vi "divide.vi"(8 "error in (no error)":errorcluster, 9 "divisor":refnum<class "Image.lvclass">, 10 "divisor":dbl=1.0, 11 "Image in":refnum<class "Image.lvclass">) -> (0 "error out":errorcluster, 3 "Image out":refnum<class "Image.lvclass">)   [LabVIEW 2010, in "Image.lvclass"]
uses:
  Image.lvclass
  storage_mode.ctl
  ErrorController/ErrorController/class_data.vi
  <vilib>/vision/NI_Vision_Development_Module.lvlib
  ErrorController/ErrorController/ErrorController.lvclass
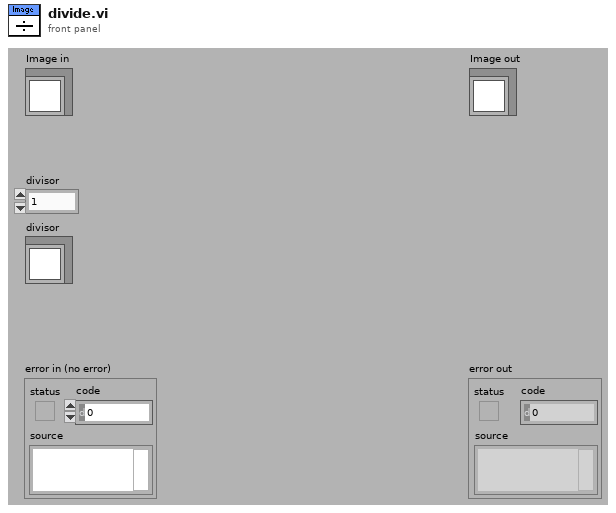
[diagram p1: front panel]
types:
  T1 = typedef "Image.lvclass/storage_mode.ctl" = enum16{"RAM", "disk"}
  T2 = typedef "IMAQ Image.ctl" = refnum<image>
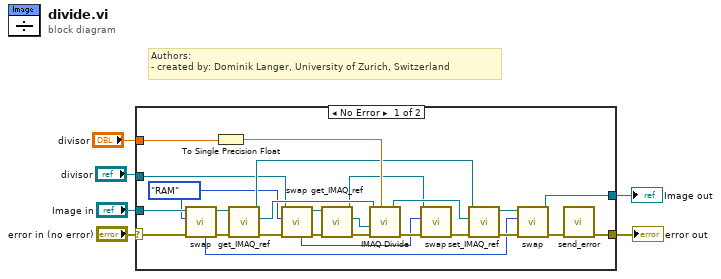
[diagram p0: block diagram]
diagram:
  # "Authors: \n- created by: Dominik Langer, University of Zurich, Switzerland"
  n1 = case shown="No Error" "error in (no error)" {
    selector: "error in (no error)" -> [w30 w34]
    tunnel: [w7 w34] -> w5
    tunnel: [w21 w33] -> w3
    tunnel: "Image in" -> [w29 w33]
    tunnel: "divisor" -> [w31 _]
    tunnel: "divisor" -> [w18 _]
    frame No Error {
      w17 = storage_mode."RAM" ("storage type target")
      n2 = call-dynamic "swap.vi"("error in (no error)"=w30, "storage type target"=w17, "Image in"=w29) -> ("error out"=w27:errorcluster, "Image out"=w28:refnum<class "Image.lvclass">, "previous storage mode"=w20:T1)  [unwired: 6 out]
      n3 = To Single Precision Float(number=w31) -> (single precision float=w32:sgl)
      n4 = call-dynamic "get_IMAQ_ref.vi"("error in (no error)"=w27, "Image.lvclass in"=w28) -> ("error out"=w19:errorcluster, "Image"=w26:T2, "Image.lvclass out"=w24:refnum<class "Image.lvclass">)  [unwired: 7 out]
      n5 = call-dynamic "swap.vi"("error in (no error)"=w19, "storage type target"=w17, "Image in"=w18) -> ("error out"=w16:errorcluster, "Image out"=w14:refnum<class "Image.lvclass">, "previous storage mode"=w10:T1)  [unwired: 6 out]
      n6 = call-dynamic "get_IMAQ_ref.vi"("error in (no error)"=w16, "Image.lvclass in"=w14) -> ("error out"=w15:errorcluster, "Image"=w13:T2, "Image.lvclass out"=w9:refnum<class "Image.lvclass">)  [unwired: 7 out]
      n7 = call "IMAQ Divide"("Image Src A"=w26, "Constant"=w32, "Image Src B"=w13, "error in (no error)"=w15) -> ("Image Dst Out"=w22:T2, "error out"=w12:errorcluster)  [unwired: 2 in, 1 out]
      n8 = call-dynamic "swap.vi"("error in (no error)"=w12, "storage type target"=w10, "Image in"=w9) -> ("error out"=w11:errorcluster)  [unwired: 8 out]
      n9 = call-dynamic "set_IMAQ_ref.vi"("error in (no error)"=w11, "Image"=w22, "Image.lvclass in"=w24) -> ("error out"=w23:errorcluster, "Image.lvclass out"=w25:refnum<class "Image.lvclass">)  [unwired: 7 out]
      n10 = call-dynamic "swap.vi"("error in (no error)"=w23, "storage type target"=w20, "Image in"=w25) -> ("error out"=w8:errorcluster, "Image out"=w21:refnum<class "Image.lvclass">)  [unwired: 7 out]
      n11 = call "send_error.vi"("error in (no error)"=w8) -> ("error out"=w7:errorcluster)  [unwired: 10 in]
    }
    frame Error {
    }
  }
  "error out" <- w5
  "Image out" <- w3
